vi "Initialize.vi"(8 "error in (no error)":errorcluster, 10 "Connection String":string, 11 "MicronServer in":refnum<class "GRPCService.lvclass">) -> (0 "error out":errorcluster, 2 "MessageUserEvent":refnum<user-event>, 3 "MicronServer out":refnum<class "GRPCService.lvclass">)   [LabVIEW 2019, in "GRPCServer.lvlib" / "GRPCService.lvclass"]
uses:
  GRPCService.lvclass
  Base/Server/Message/MessageBase.lvclass
  Base/Server/Service/ServiceBase.lvclass
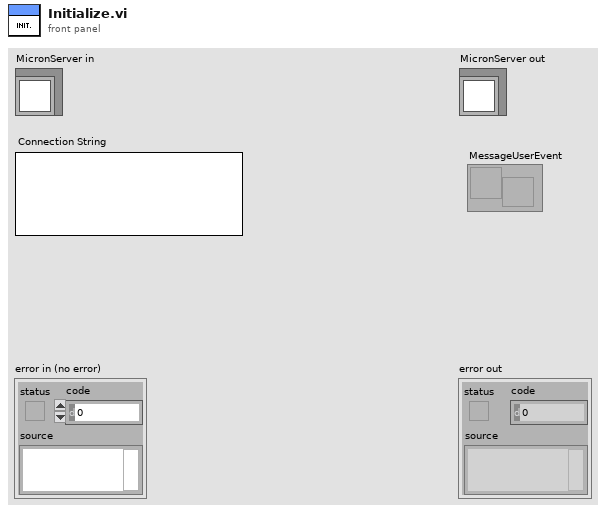
[diagram p1: front panel]
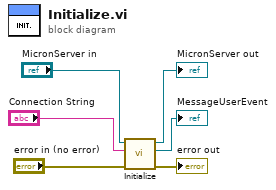
[diagram p0: block diagram]
diagram:
  n1 = call-parent "Initialize.vi"("error in (no error)"="error in (no error)", "Connection String"="Connection String", "MicronServer in"="MicronServer in") -> ("error out"=→"error out":errorcluster, "MessageUserEvent"=→"MessageUserEvent":refnum<user-event>, "MicronServer out"=→"MicronServer out":refnum<class "GRPCService.lvclass">)  [unwired: 6 in]
